vi "SQLCloseCursor.vi"(4 "error in (no error)":errorcluster, 7 "InputHandle":i32) -> (0 "error out":errorcluster, 3 "OutputHandle":i32)   [LabVIEW 2011]
doc: "Ferme le curseur de la requête"
uses:
  Odbc32.dll
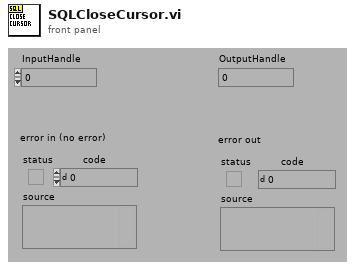
[diagram p1: front panel]
types:
  T1 = enum16{"NOPE", "SQL_HANDLE_ENV", "SQL_HANDLE_DBC", "SQL_HANDLE_STMT", "SQL_HANDLE_DESC"}
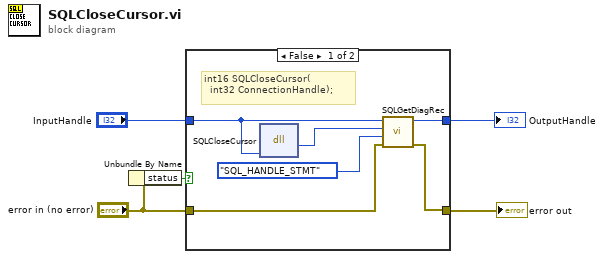
[diagram p0: block diagram]
diagram:
  n1 = Unbundle By Name("error in (no error)") -> ("status"=w3:bool)
  n2 = case shown="False" w3 {
    tunnel: "InputHandle" -> [w8 w12]
    tunnel: "error in (no error)" -> [w10 w13]
    tunnel: [w9 w13] -> w2
    tunnel: [w7 w12] -> w1
    frame False {
      # "int16 SQLCloseCursor(\n  int32 ConnectionHandle);"
      n3 = dll-call lib="Odbc32.dll" fn="SQLCloseCursor"("ConnectionHandle"=w8) -> (w11:i16)  [unwired: 4 in, 2 out]
      n4 = call "SQLGetDiagRec.vi"("error in (no error)"=w10, "HandleType"=T1."SQL_HANDLE_STMT", "Status (SQL_SUCCESS=0)"=w11, "Input Handle"=w8) -> ("error out"=w9:errorcluster, "Output Handle"=w7:i32)  [unwired: 2 out]
    }
    frame True {
    }
  }
  "OutputHandle" <- w1
  "error out" <- w2
